vi "HV_Onstate_Multi.vi"(8 "Power":bool[](array[boolean]), 11 "Channel":string[](array[string])) -> (3 "Output":string[](array[string]))   [LabVIEW 2019]
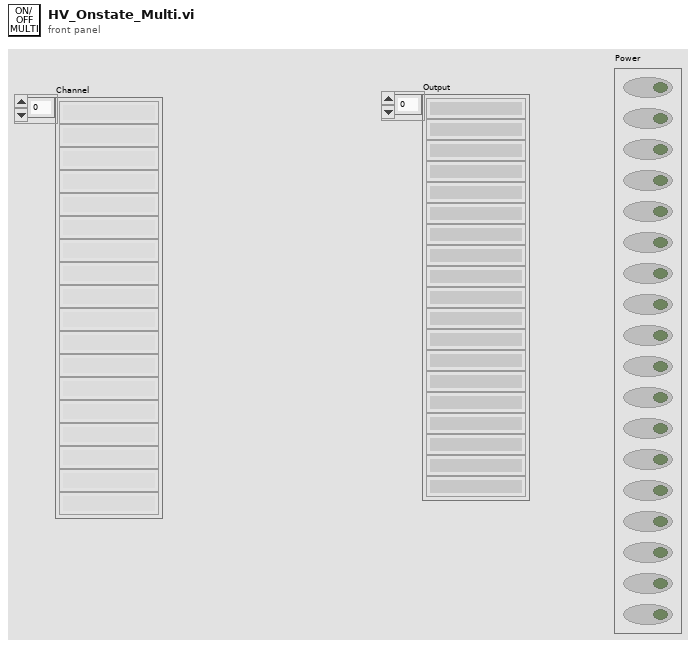
[diagram p1: front panel]
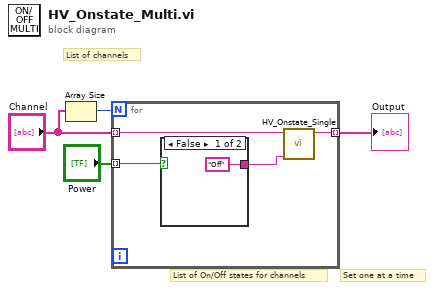
[diagram p0: block diagram]
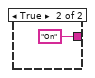
[diagram p2: hidden frame]
diagram:
  # "Set one at a time"
  # "List of On/Off states for channels"
  # "List of channels"
  n1 = Array Size(array="Channel") -> (size(s)=w3:i32)
  n2 = for {
    N: w3 -> [_]
    tunnel: "Channel" -> [w8] mode=indexing
    tunnel: "Power" -> [w6] mode=indexing
    tunnel: [w7] -> w2 mode=indexing
    n3 = case shown="False" w6 {
      tunnel: ["Off" "On"] -> w5
      frame False {
      }
      frame True {
      }
    }
    n4 = call "HV_Onstate_Single.vi"("On/Off"=w5, "Channel"=w8) -> ("standard output"=w7:string)  [unwired: 9 in]
  }
  "Output" <- w2
